vi "Initialize.vi"(8 "error in":errorcluster, 11 "NI name":string) -> (0 "error out":errorcluster, 3 "Modbus master out":refnum<class "Modbus Master.lvclass">)   [LabVIEW 2023, in "RS485.lvlib"]
uses:
  RS485.lvlib
  <vilib>/NI/Modbus Library/API/Master/Modbus Master.lvclass
  <vilib>/NI/Modbus Library/API/Wrapper/Create Serial Master.vi
  <vilib>/NI/Modbus Library/API/Wrapper/API Main.lvlib
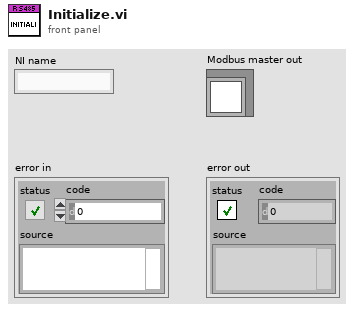
[diagram p1: front panel]
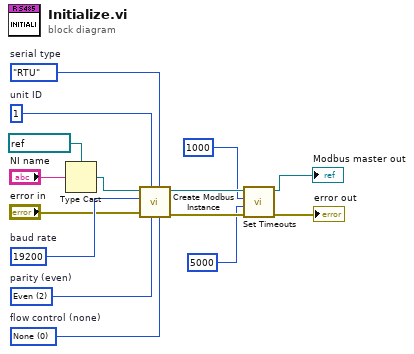
[diagram p0: block diagram]
diagram:
  w15 = u8 1  # unit ID
  w10 = u16 0 items=["None", "XON/XOFF", "RTS/CTS", "XON/XOFF & RTS/CTS", "DTR/DSR", "XON/XOFF & DTR/DSR"]  # flow control (none)
  w11 = u16 2 items=["None", "Odd", "Even", "Mark", "Space"]  # parity (even)
  w14 = u32 19200  # baud rate
  w13 = enum16{"RTU", "ASCII"}."RTU"  # serial type
  n1 = Type Cast(type=refnum<visa-resource-name> "COM5" ("VISA resource name"), x="NI name") -> (*(type *) &x=w1:refnum<visa-resource-name>)
  n2 = call-poly <vilib>:"Create Modbus Instance.vi"("flow control (none)"=w10, "serial type"=w13, "parity (even)"=w11, "unit ID"=w15, "error in"="error in", "baud rate"=w14, "VISA resource name"=w1) -> ("error out"=w8:errorcluster, "serial master instance"=w9:refnum<class "Modbus Master.lvclass">)  [unwired: 3 in]
  n3 = call <vilib>:"Set Timeouts.vi"("error in"=w8, "write operation timeout"=5000, "read operation timeout"=1000, "Modbus master in"=w9) -> ("error out"=→"error out":errorcluster, "Modbus master out"=→"Modbus master out":refnum<class "Modbus Master.lvclass">)  [unwired: 6 in]
